vi "NXT arbiter demo A.vi"() -> ()   [LabVIEW 2012]
panel:
  in  "Distance array":i16[](array[numeric])=[800, 800, 800, 800, 800, 700, 600, 500, 500, 600, 700, 800, 800, 800, 800, 800]
  in  "FB Arbiter \nVelocity":i16=7
  out "Index":i16
  in  "stop":bool
  in  "FB weight":dbl=0.6
  out "Tug array":cluster{i32, i32, "Normalized\nArray":i16[]}(graph)
  in  "Local Heading":i16 step=1
  out "Motor":u16
  out "Rudder":u16
  out "Right turn?":bool
  out "Arbiter\nvelocity":i16
  out "Arbiter Heading":i16
  out "Average of all":cluster{i32, i32, "Obs array":i16[]}[](graph)
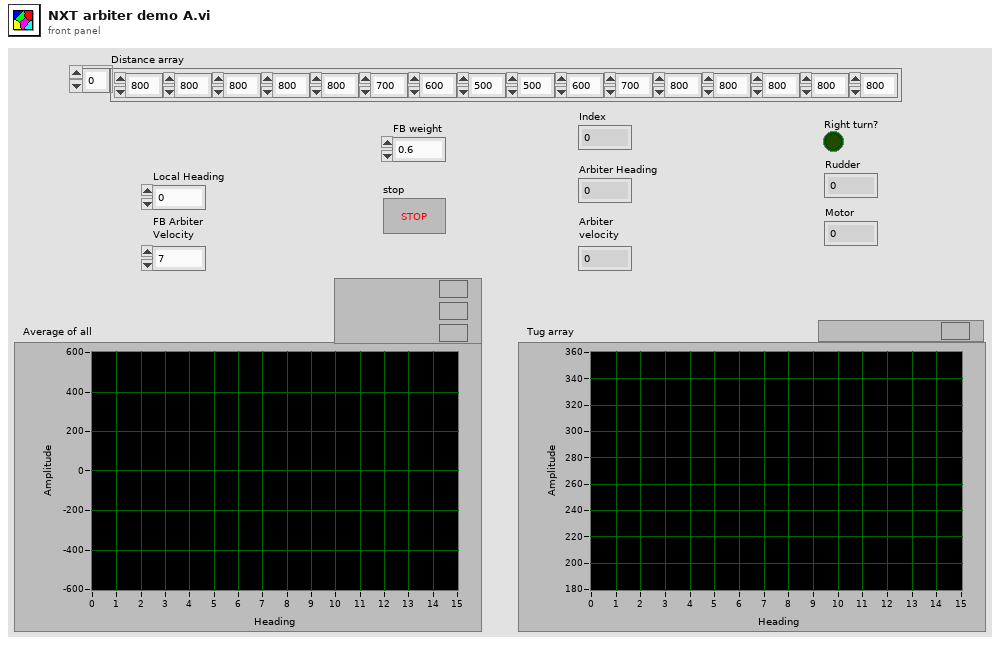
[diagram p1: front panel]
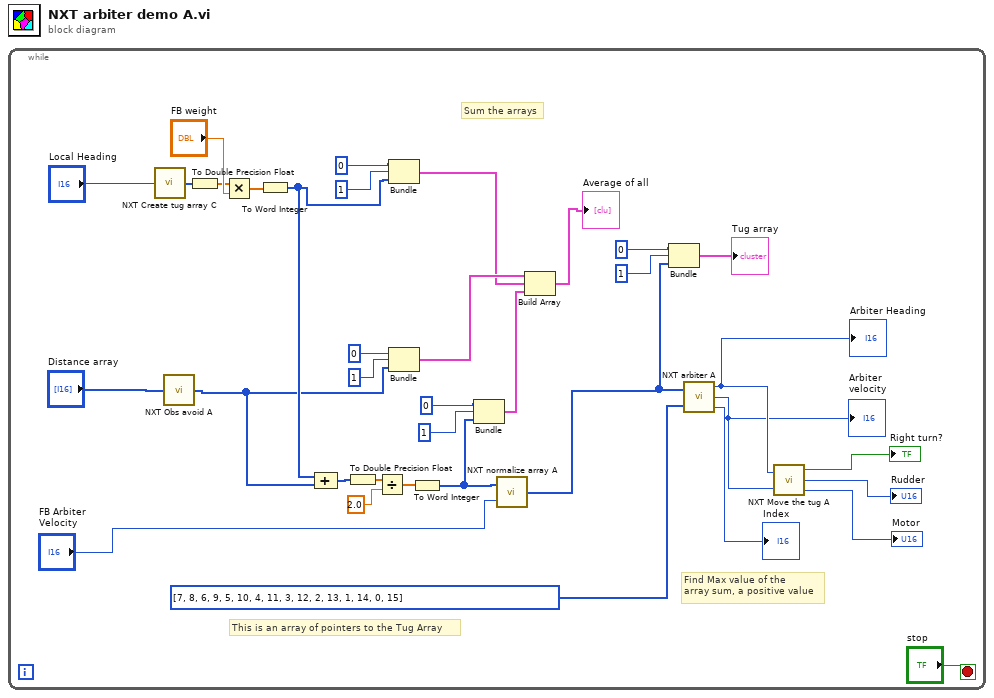
[diagram p0: block diagram]
diagram:
  n1 = while {
    stop <- "stop" stop-if-true
    # "This is an array of pointers to the Tug Array"
    # "Find Max value of the\narray sum, a positive value"
    # "Sum the arrays"
    n2 = call "NXT Create tug array C.vi"("Local Heading"="Local Heading") -> ("FB array"=w6:i16[])  [unwired: 2 in]
    n3 = call "NXT Obs avoid A.vi"("Distance array"="Distance array") -> ("Obs array"=w2:i16[])
    n4 = To Double Precision Float(number=w6) -> (double precision float=w15:dbl[])
    n5 = Multiply(x=w15, y="FB weight") -> (x*y=w28:dbl[])
    n6 = To Word Integer(number=w28) -> (16bit integer=w7:i16[])
    n7 = Compound Arithmetic op=ADD(w7, w2) -> (w8:i16[])
    n8 = To Double Precision Float(number=w8) -> (double precision float=w14:dbl[])
    n9 = Divide(x=w14, y=2.0) -> (x/y=w19:dbl[])
    n10 = Bundle(0, 1, w7) -> (w13:cluster{i32, i32, i16[]})  [unwired: 1 in]
    n11 = Bundle(0, 1, "Obs array"=w2) -> (w18:cluster{i32, i32, "Obs array":i16[]})  [unwired: 1 in]
    n12 = To Word Integer(number=w19) -> (16bit integer=w11:i16[])
    n13 = Bundle(0, 1, w11) -> (w12:cluster{i32, i32, i16[]})  [unwired: 1 in]
    n14 = call "NXT normalize array A.vi"("FB Arbiter\nVelocity"="FB Arbiter \nVelocity", "Tug array"=w11) -> ("Normalized\nArray"=w9:i16[])
    n15 = Build Array(w18, w13, w12) -> (→"Average of all":cluster{i32, i32, "Obs array":i16[]}[])
    n16 = Bundle(0, 1, "Normalized\nArray"=w9) -> (→"Tug array":cluster{i32, i32, "Normalized\nArray":i16[]})  [unwired: 1 in]
    n17 = call "NXT arbiter A.vi"("Tug array"=w9, "Array angle\npointers"=i16[] [7, 8, 6, 9, 5, 10, 4, 11, 3, 12, 2, 13, 1, 14, 0, 15] ("Array angle\npointers")) -> ("Arbiter Heading"=w24:i16, "Arbiter\nvelocity"=w23:i16, "Index"=→"Index":i16)
    "Arbiter Heading" <- w24
    "Arbiter\nvelocity" <- w23
    n18 = call "NXT Move the tug A.vi"("Arbiter Heading"=w24, "Desired Speed"=w23) -> ("Right turn?"=→"Right turn?":bool, "Rudder"=→"Rudder":u16, "Motor"=→"Motor":u16)
  }
